vi "Write Emergency.vi"(8 "error in (no error)":errorcluster, 10 "Emergency":bool, 11 "Display Console in":refnum<class "Display Console.lvclass">) -> (0 "error out":errorcluster, 3 "Display Console out":refnum<class "Display Console.lvclass">)   [LabVIEW 2019, in "Display Console Actor.lvlib" / "Display Console.lvclass"]
uses:
  Display Console.lvclass
  Display Console.lvclass/Display Console.ctl
  Abstract Display Console Actor/Abstract Display Console Actor/Abstract Display Console.lvclass
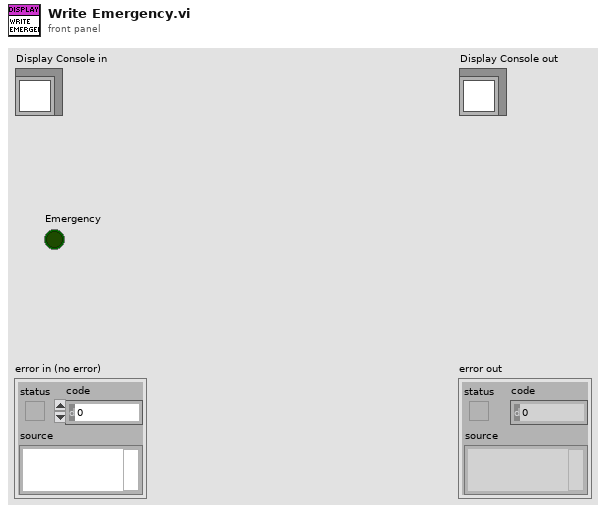
[diagram p1: front panel]
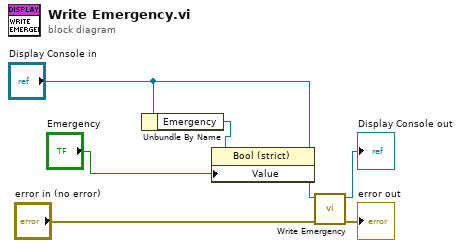
[diagram p0: block diagram]
diagram:
  n1 = Unbundle By Name("Display Console in") -> ("Emergency"=w2:refnum<vi>)
  n2 = property class="Bool (strict)"(reference=w2, "Value"="Emergency") -> ()  [unwired: 1 in, 2 out]
  n3 = call-parent "Write Emergency.vi"("error in (no error)"="error in (no error)", "Abstract Display Console in"="Display Console in") -> ("error out"=→"error out":errorcluster, "Abstract Display Console out"=→"Display Console out":refnum<class "Display Console.lvclass">)  [unwired: 8 in]
